vi "Receive_Message.vi"(8 "error in (no error)":errorcluster, 11 "connection ID IN":refnum<k5>) -> (0 "error out (no error)":errorcluster, 2 "msg OUT":T1={"message data"=variant, "message type"=enum."Stop"}, 3 "connection ID OUT":refnum<k5>)   [LabVIEW 2013]
uses:
  Messages.ctl
  messageTypes.ctl
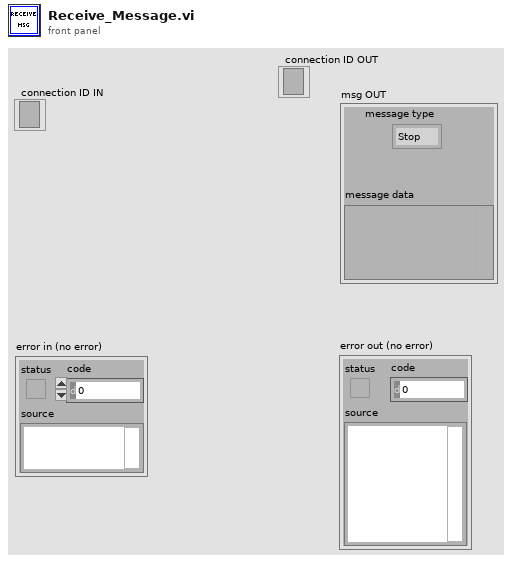
[diagram p1: front panel]
types:
  T1 = typedef "Messages.ctl" = cluster{"message data":variant, "message type":T2}
  T2 = typedef "messageTypes.ctl" = enum16{"Speeds", "Stop", "PolarCoordinates", "Gains", "Setpoints"}
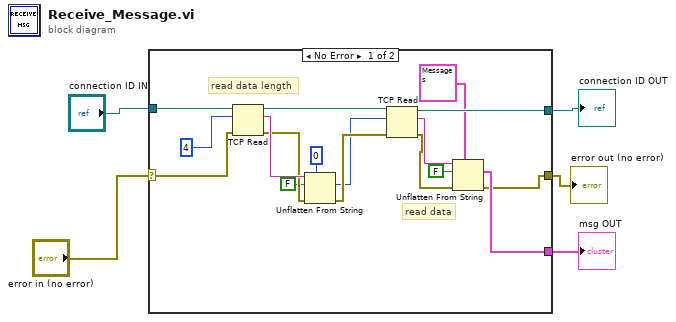
[diagram p0: block diagram]
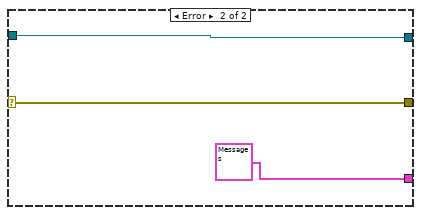
[diagram p2: hidden frame]
diagram:
  n1 = case shown="No Error" "error in (no error)" {
    selector: "error in (no error)" -> [w20 w25]
    tunnel: [w9 w25] -> w4
    tunnel: "connection ID IN" -> [w21 w24]
    tunnel: [w13 w24] -> w1
    tunnel: [w10 T1 {"message data"=variant, "message type"=enum."Stop"} ("message")] -> w2
    frame No Error {
      # "read data"
      # "read data length"
      n2 = TCP Read(connection ID=w21, bytes to read=4, error in (no error)=w20) -> (connection ID out=w18:refnum<k5>, data out=w19:string, error out=w17:errorcluster)  [unwired: 2 in]
      n3 = Unflatten From String(type=0, binary string=w19, data includes array or string size? (T)=FALSE, error in (no error)=w17) -> (value=w15:i32, error out=w16:errorcluster)  [unwired: 1 in, 1 out]
      n4 = TCP Read(connection ID=w18, bytes to read=w15, error in (no error)=w16) -> (connection ID out=w13:refnum<k5>, data out=w12:string, error out=w11:errorcluster)  [unwired: 2 in]
      n5 = Unflatten From String(type=T1 {"message data"=variant, "message type"=enum."Setpoints"} ("message"), binary string=w12, data includes array or string size? (T)=FALSE, error in (no error)=w11) -> (value=w10:T1, error out=w9:errorcluster)  [unwired: 1 in, 1 out]
    }
    frame Error {
    }
  }
  "error out (no error)" <- w4
  "msg OUT" <- w2
  "connection ID OUT" <- w1
